vi "cg_fid_V1.2.2.vi"() -> ()   [LabVIEW 2011]
panel:
  out "time string":string
  out "date string":string
  out "Elapsed Time (s)":dbl
  in  "stop":bool
  in  "error IO":errorcluster
  in  "Number of Injections":dbl
  out "Start Indicator":bool
  in  "start chromat":bool
  in  "Abort Chrom":bool
  out "FID":cluster{"value":dbl}(graph)
  out "Temp History":cluster{"value":dbl}(graph)
  out "Time (min)":dbl
  out "Counter":i32
  in  "Stop Time (min)":dbl=15.0
  out "Time has Elapsed":bool
  in  "Start Button":bool
  out "TCD":dbl(graph)
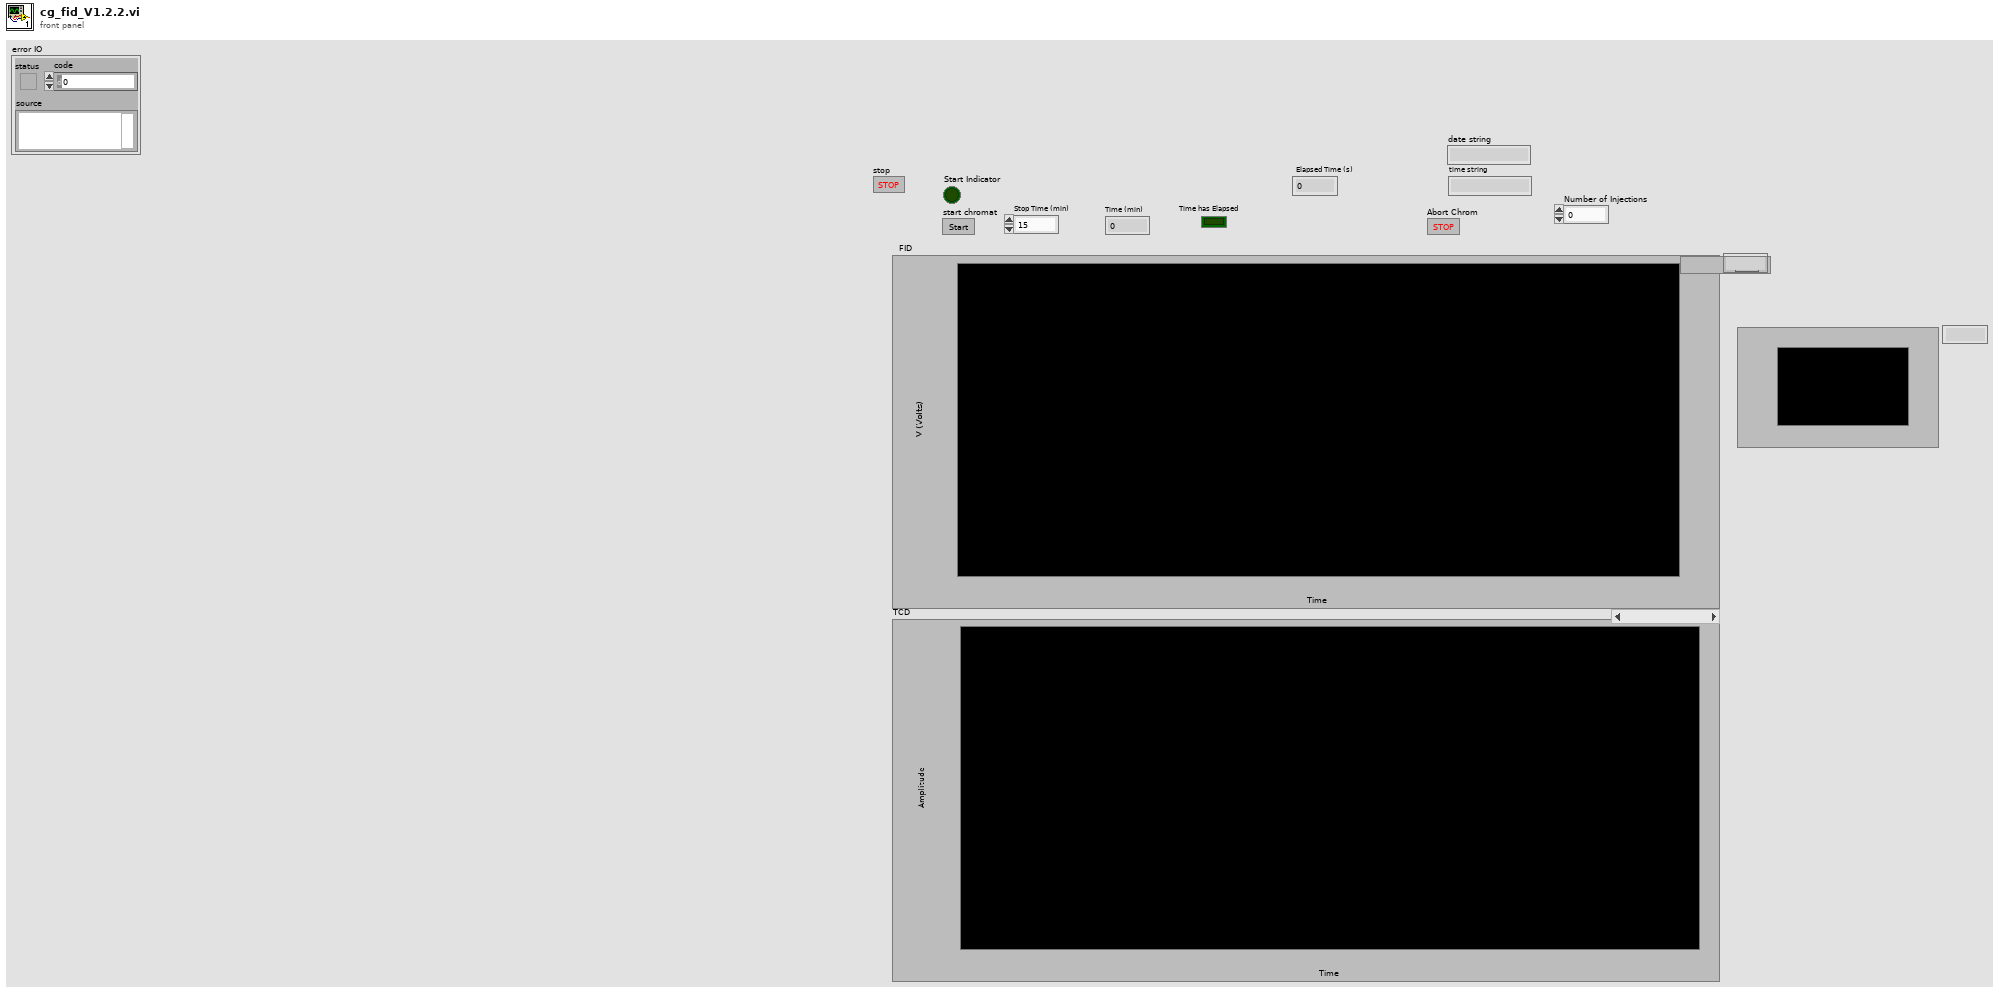
[diagram p1: front panel]
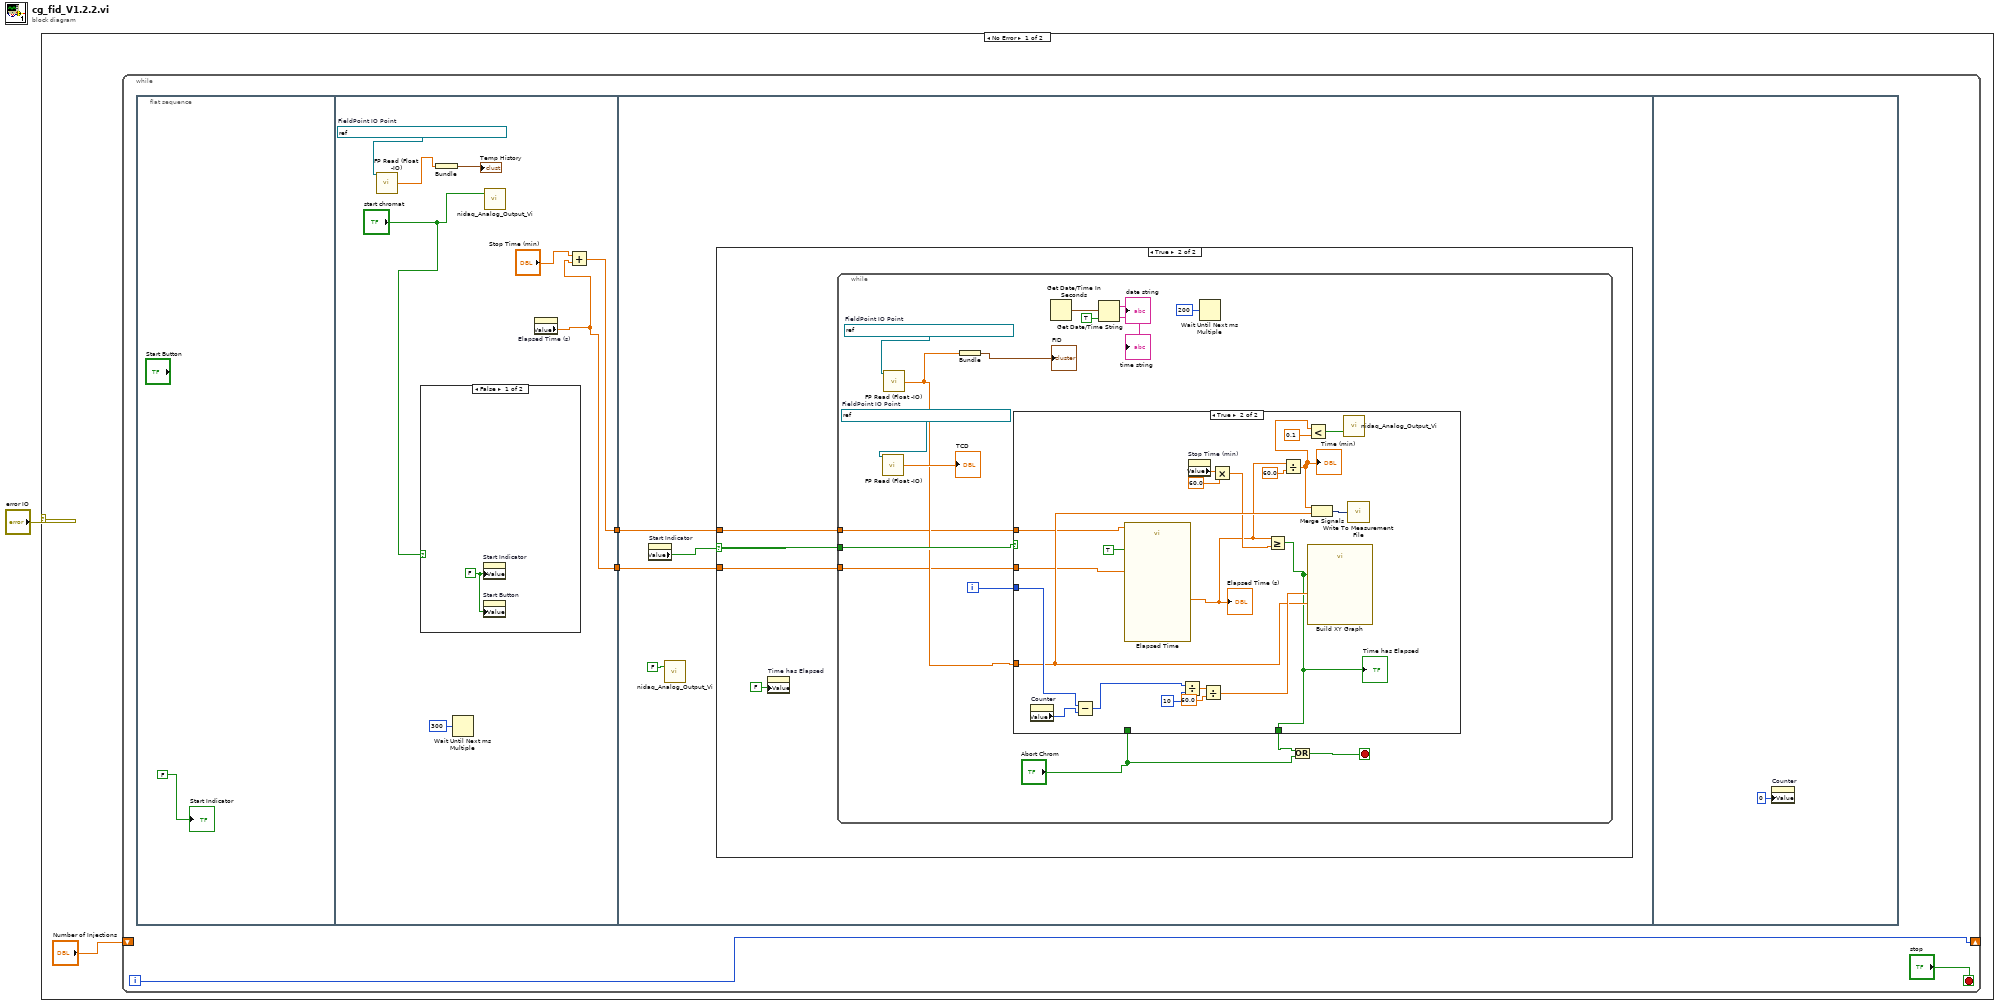
[diagram p0: block diagram]
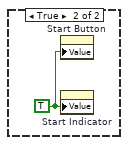
[diagram p2: hidden frame]
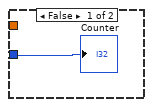
[diagram p4: hidden frame]
diagram:
  n1 = case shown="No Error" "error IO" {
    frame No Error {
      n2 = while {
        shift-right: [w6] -> _
        shift-left: "Number of Injections" -> [_]
        i -> [w6]
        stop <- "stop" stop-if-true
        n3 = flat-sequence {
          tunnel: [w8] -> w4
          tunnel: [w9] -> w3
          tunnel: w4 -> [w19]
          tunnel: w3 -> [w18]
          frame #0 {
            "Start Indicator" <- FALSE
          }
          frame #1 {
            w14 = refnum<k21> "FieldPoint\\cfp2220\\cFP-AI-110 @4\\Channel 0"  # FieldPoint IO Point
            n4 = call <vilib>:"FP Read (Float -IO).vi"("FieldPoint IO Point In"=w14) -> ("value"=w13:dbl)  [unwired: 11 in, 3 out]
            n5 = case shown="False" "start chromat" {
              frame False {
                w16 = FALSE ("Start Button")
                n6 = property on="Start Indicator" class="Bool (strict)"("Value"=w16) -> ()  [unwired: 2 in, 2 out]
                n7 = property on="Start Button" class="Bool (strict)"("Value"=w16) -> ()  [unwired: 2 in, 2 out]
              }
              frame True {
                w17 = TRUE ("Start Button")
                n8 = property on="Start Button" class="Bool (strict)"("Value"=w17) -> ()  [unwired: 2 in, 2 out]
                n9 = property on="Start Indicator" class="Bool (strict)"("Value"=w17) -> ()  [unwired: 2 in, 2 out]
              }
            }
            n10 = Bundle("value"=w13) -> (→"Temp History":cluster{"value":dbl})  [unwired: 1 out]
            n11 = Wait Until Next ms Multiple(millisecond multiple=u32 300) -> ()  [unwired: 1 out]
            n12 = call "nidaq_Analog_Output_Vi.vi"("start chromat"="start chromat") -> ()  [unwired: 2 in]
            n13 = property on="Elapsed Time (s)" class="DigNum (strict)"() -> ("Value"=w8:dbl)  [unwired: 2 in, 2 out]
            n14 = Add(x="Stop Time (min)", y=w8) -> (x+y=w9:dbl)
          }
          frame #2 {
            n15 = property on="Start Indicator" class="Bool (strict)"() -> ("Value"=w21:bool)  [unwired: 2 in, 2 out]
            n16 = call "nidaq_Analog_Output_Vi.vi"("start chromat"=FALSE) -> ()  [unwired: 2 in]
            n17 = case shown="True" w21 {
              selector: w21 -> [_ w25]
              tunnel: w19 -> [_ w23]
              tunnel: w18 -> [_ w22]
              frame False {
              }
              frame True {
                n18 = property on="Time has Elapsed" class="Bool (strict)"("Value"=FALSE ("Time has Elapsed")) -> ()  [unwired: 2 in, 2 out]
                n19 = while {
                  tunnel: w25 -> [w36]
                  tunnel: w23 -> [w31]
                  tunnel: w22 -> [w30]
                  i -> [w38]
                  stop <- w33 stop-if-true
                  w41 = refnum<k21> "FieldPoint\\cfp2220\\cFP-AI-110 @4\\Channel 2"  # FieldPoint IO Point
                  w42 = refnum<k21> "FieldPoint\\cfp2220\\cFP-AI-110 @4\\Channel 0"  # FieldPoint IO Point
                  n20 = call <vilib>:"FP Read (Float -IO).vi"("FieldPoint IO Point In"=w41) -> ("value"=→"TCD":dbl)  [unwired: 11 in, 3 out]
                  n21 = call <vilib>:"FP Read (Float -IO).vi"("FieldPoint IO Point In"=w42) -> ("value"=w34:dbl)  [unwired: 11 in, 3 out]
                  n22 = Bundle("value"=w34) -> (→"FID":cluster{"value":dbl})  [unwired: 1 out]
                  n23 = case shown="True" w36 {
                    tunnel: w34 -> [_ w54]
                    tunnel: w38 -> [w43 w60]
                    tunnel: [_ w48] -> w35
                    tunnel: "Abort Chrom" -> [_ _]
                    tunnel: w31 -> [_ w50]
                    tunnel: w30 -> [_ w49]
                    frame False {
                      "Counter" <- w43
                    }
                    frame True {
                      n24 = property on="Counter" class="DigNum (strict)"() -> ("Value"=w59:i32)  [unwired: 2 in, 2 out]
                      n25 = Subtract(x=w60, y=w59) -> (x-y=w61:i32)
                      n26 = call "Elapsed Time"("Time Target (s)"=w49, "Auto Reset"=TRUE, "Set Start Time (s)"=w50) -> ("Elapsed Time (s)"=w44:dbl)  [unwired: 9 in, 7 out]
                      "Elapsed Time (s)" <- w44
                      n27 = Divide(x=w61, y=10) -> (x/y=w63:dbl)
                      n28 = property on="Stop Time (min)" class="DigNum (strict)"() -> ("Value"=w47:dbl)  [unwired: 2 in, 2 out]
                      n29 = Divide(x=w63, y=60.0) -> (x/y=w58:dbl)
                      n30 = Multiply(x=w47, y=60.0) -> (x*y=w45:dbl)
                      n31 = Greater Or Equal?(x=w44, y=w45) -> (x >= y?=w48:bool)
                      "Time has Elapsed" <- w48
                      n32 = Divide(x=w44, y=60.0) -> (x/y=w51:dbl)
                      "Time (min)" <- w51
                      n33 = Less?(x=w51, y=0.1) -> (x < y?=w53:bool)
                      n34 = call "Build XY Graph"("Enable"=w48, "Y Input"=w54, "X Input"=w58) -> ()  [unwired: 2 in, 7 out]
                      n35 = Merge Signals(w51, w54) -> (w56:dynamicdata)
                      n36 = call "nidaq_Analog_Output_Vi.vi"("start Solenoide Valve"=w53) -> ()  [unwired: 2 in]
                      n37 = call "Write To Measurement File"("Signals"=w56) -> ()  [unwired: 16 in, 3 out]
                    }
                  }
                  n38 = Get Date/Time In Seconds() -> (seconds since 1Jan1904=w27:timestamp)
                  n39 = Get Date/Time String(seconds (now)=w27, want seconds? (F)=TRUE) -> (date string=→"date string":string, time string=→"time string":string)  [unwired: 1 in]
                  n40 = Wait Until Next ms Multiple(millisecond multiple=u32 200) -> ()  [unwired: 1 out]
                  n41 = Or(x=w35, y="Abort Chrom") -> (x .or. y?=w33:bool)
                }
              }
            }
          }
          frame #3 {
            n42 = property on="Counter" class="DigNum (strict)"("Value"=0 ("Numeric")) -> ()  [unwired: 2 in, 2 out]
          }
        }
      }
    }
    frame Error {
    }
  }
